vi "StateTriggerConfigure.vi"(5 "Identifier":string, 6 "Filter":string, 7 "Detection (High)":i32(ring) items=["High", "Low", "Rise", "Fall"], 8 "error in (no error)":errorcluster {"code" format="%.0x"}, 9 "Enabled (Off)":bool, 10 "RepCapIdentifier":string="StateTrigger_LAN0" caption="RepCapIdentifier (StateTrigger_LAN0)", 11 "instrument handle":refnum<k15>) -> (0 "error out":errorcluster {"code" format="%.0x"}, 3 "instrument handle out":refnum<k15>)   [LabVIEW 2009, in "Keysight XSAn.lvlib"]
doc: "Allows the configuration of some of the parameters from a single command.\n\nSupported Models : M9290A, M9420A, M9421A, N9000A, N9000B, N9010A, N9010B, N9020A, N9020B, N9030A, N9030B, N9038A, N9040B, N9041B, SPN9003A, SPN9026A"
uses:
  <instrlib>/Keysight XSAn/Keysight XSAn.lvlib
  AgXSAn.dll
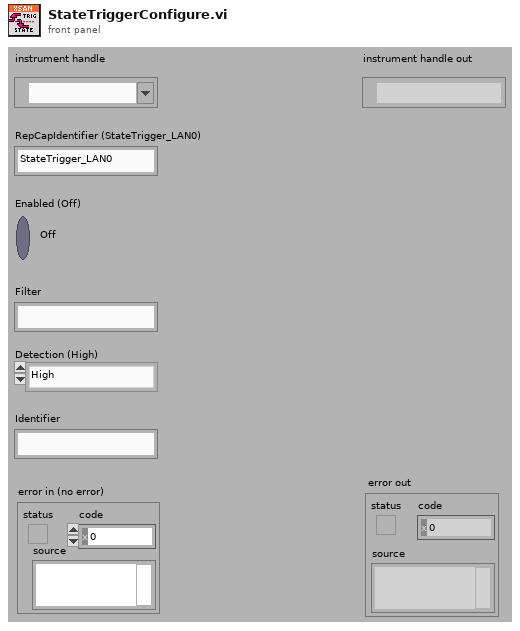
[diagram p1: front panel]
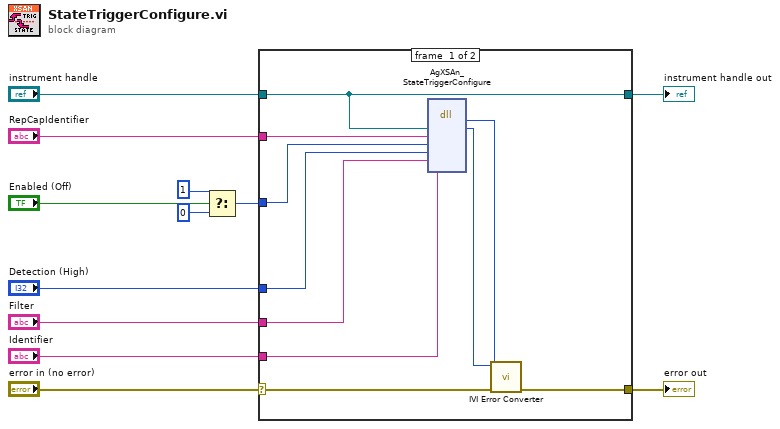
[diagram p0: block diagram]
diagram:
  n1 = Select(t=u16 1, s="Enabled (Off)", f=u16 0) -> (s? t:f=w5:u16)
  n2 = case shown="No Error" "error in (no error)" {
    selector: "error in (no error)" -> [w20 w24]
    tunnel: [w19 w24] -> w12
    tunnel: "instrument handle" -> [w13 w23]
    tunnel: "RepCapIdentifier" -> [w18 _]
    tunnel: w5 -> [w17 _]
    tunnel: "Detection (High)" -> [w16 _]
    tunnel: "Filter" -> [w15 _]
    tunnel: "Identifier" -> [w14 _]
    tunnel: [w13 w23] -> w1
    frame #0 {
      n3 = dll-call lib="AgXSAn**.dll" fn="AgXSAn_StateTriggerConfigure"("Vi"=w13, "RepCapIdentifier"=w18, "Enabled"=w17, "Detection"=w16, "Filter"=w15, "Identifier"=w14) -> (w21:i32, "Vi"=w22:u32)  [unwired: 8 in, 2 out]
      n4 = call <instrlib>:"IVI Error Converter.vi"("error in (no error)"=w20, "IVI error code (0)"=w21, "instrument handle"=w22) -> ("error out"=w19:errorcluster)  [unwired: 7 in, 1 out]
    }
    frame #1 {
    }
  }
  "error out" <- w12
  "instrument handle out" <- w1
